vi "Update Grp Mem MCLB.vi"(8 "error in":errorcluster, 10 "Item Names":string[][](array[string]), 11 "FP Ctrls":refnum<class "FP Controls.lvclass">) -> (0 "error out":errorcluster, 3 "FP Ctrls":refnum<class "FP Controls.lvclass">)   [LabVIEW 2018, in "Configuration Grandmaster.lvlib" / "FP Controls.lvclass"]
uses:
  FP Controls.lvclass
  FP Controls.lvclass/FP Controls.ctl
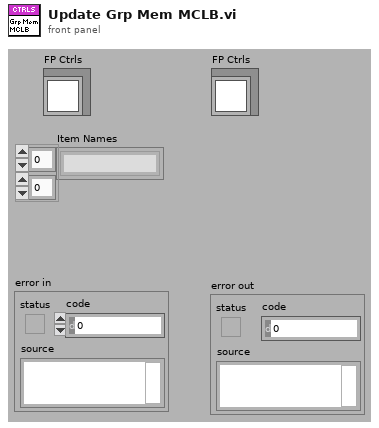
[diagram p1: front panel]
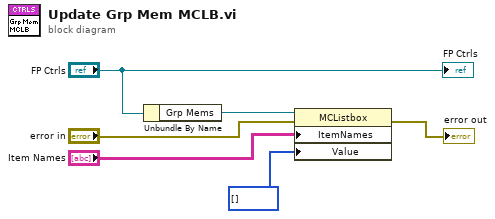
[diagram p0: block diagram]
diagram:
  n1 = Unbundle By Name("FP Ctrls") -> ("Grp Mems"=w1:refnum<vi>)
  n2 = property on="Property Node" class="MCListbox"(reference=w1, error in="error in", "ItemNames"="Item Names", "Value"=i32[] [] ("Selected Rows")) -> (error out=→"error out":errorcluster)  [unwired: 1 out]
  "FP Ctrls" <- "FP Ctrls"
